vi "Read States.vi"(8 "error in (no error)":errorcluster, 11 "KickToBestRobotTactic in":refnum<class "KickToBestRobotTactic.lvclass">) -> (0 "error out":errorcluster, 2 "States":T1=enum."Exit", 3 "KickToBestRobotTactic out":refnum<class "KickToBestRobotTactic.lvclass">)   [LabVIEW 2024, in "KickToBestRobotTactic.lvclass"]
uses:
  KickToBestRobotTactic.lvclass
  KickTOBestRobotTacticStatesEnum.ctl
  KickToBestRobotTactic.lvclass/KickToBestRobotTactic.ctl
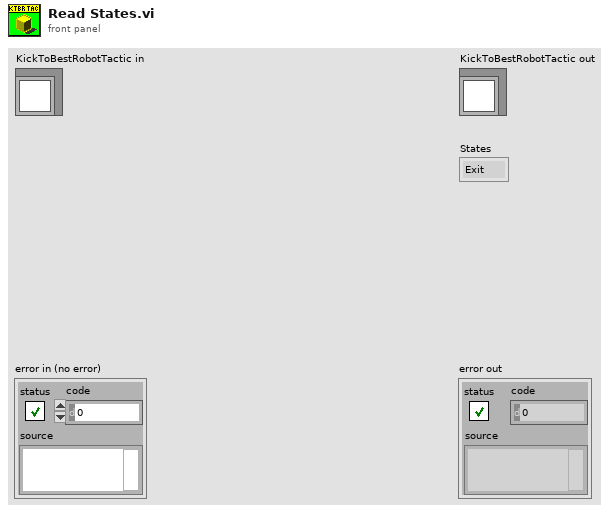
[diagram p1: front panel]
types:
  T1 = typedef "KickToBestRobotTactic.lvclass/KickTOBestRobotTacticStatesEnum.ctl" = enum16{"WaitToPass", "Pass", "Exit"}
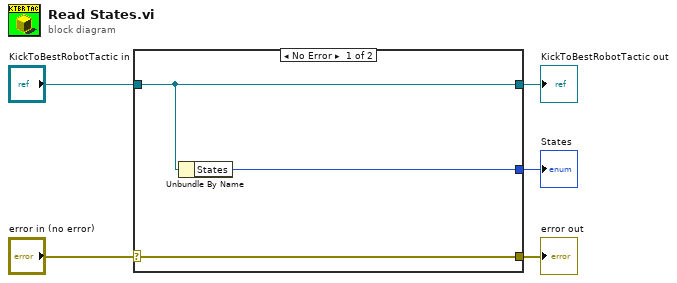
[diagram p0: block diagram]
diagram:
  n1 = case shown="No Error" "error in (no error)" {
    selector: "error in (no error)" -> [w8 w9]
    tunnel: [w8 w9] -> w4
    tunnel: [w7 w10] -> w2
    tunnel: "KickToBestRobotTactic in" -> [w7 w10]
    tunnel: [w6 _] -> w1
    frame No Error {
      n2 = Unbundle By Name(w7) -> ("States"=w6:T1)
    }
    frame Error {
    }
  }
  "error out" <- w4
  "KickToBestRobotTactic out" <- w2
  "States" <- w1
